vi "DIO Block Write.vi"(7 "Divisor":u16, 8 "DIR":bool, 9 "OUT":bool, 10 "DMA FIFO In":refnum<k21>="A.DO1 DMA", 11 "DIO Refnum":refnum<k21>="ConnectorA/DIO0") -> (1 "Timed Out?":bool, 3 "IN":bool)   [LabVIEW 2014]
uses:
  <vilib>/rvi/eio/common/nirviEmuReportErrorAndStop.vi
  <vilib>/rvi/interface/RandomDataEmulation/niFpgaRandomDataHandleErrors.vi
  <vilib>/rvi/Emulation/niFpgaProcessEmulError.vi
  <vilib>/rvi/FIFO/Fifo_Resource/nirvififoEmulationSetSize.vi
  <vilib>/rvi/DataTransferAndStorage/Container/Common/niFpgaContainerGetUniqueNameForEmu.vi
  <vilib>/rvi/FIFO/Fifo_Resource/nirviFifoEmulationQueueMgr.vi
  <instcachedir>/0/nirviFifoEmulationQueueMgr_E5CAEC123FF24DC58D834DCA3CDAA9B5.lvgen/nirviFifoEmulationQueueMgr_E5CAEC123FF24DC58D834DCA3CDAA9B5_001.vi
  <vilib>/rvi/Emulation/niFpgaEmulationIsFPGAContextNoSignature.vi
  <vilib>/rvi/errors/nirviReportUnexpectedCaseInternalError.vi
  <vilib>/rvi/errors/nirviReportUnexpectedCaseInternalError (U32).vi
  <vilib>/rvi/occurrence/nirviWaitOnOccurrenceBase.vi
  <vilib>/rvi/FIFO/Fifo_Resource/nirvififoEmulationReleaseLock.vi
  <vilib>/rvi/FIFO/Fifo_Resource/nirvififoEmulationObtainLock.vi
  <vilib>/rvi/FIFO/Fifo_Resource/nirvififoEmulationCreateLock.vi
  <vilib>/rvi/errors/niFpgaSetErrorForExecOnDevCompSimple.vi
  <vilib>/rvi/Emulation/niFpgaSctlEmulationGetInTimedLoop.vi
  <vilib>/rvi/FIFO/Fifo_Resource/nirvififoEmulationDetermineInputValidOut.vi
  <vilib>/rvi/DataTransferAndStorage/Container/Common/niFpgaContainerExecOnDevCompGetState.vi
  <vilib>/rvi/DataTransferAndStorage/Container/XNode/niFpgaContainer.xnode
  <vilib>/rvi/FIFO/Fifo_Resource/niFpgaFifoEmulationRefIn.vi
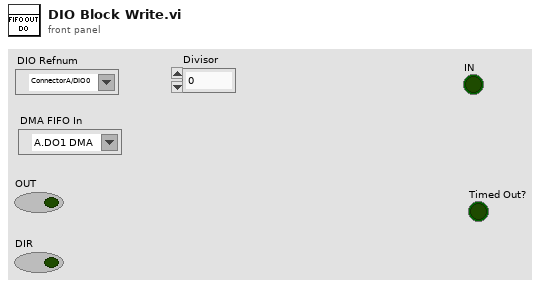
[diagram p1: front panel]
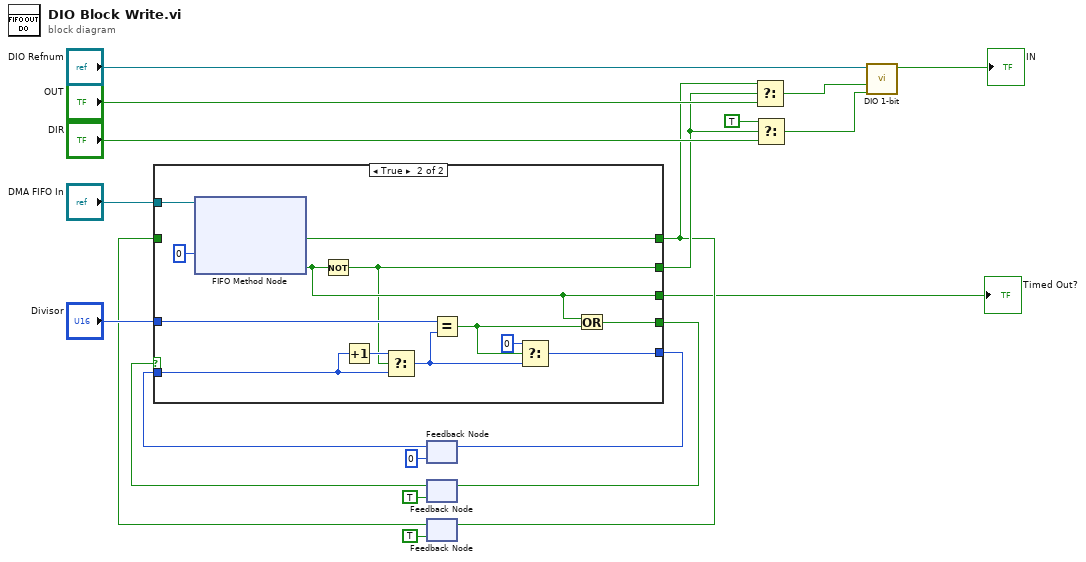
[diagram p0: block diagram]
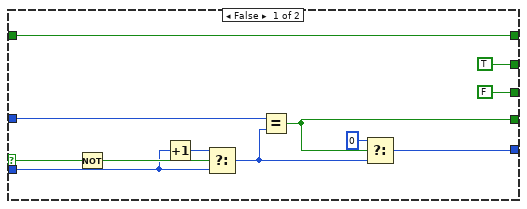
[diagram p2: hidden frame]
diagram:
  n1 = feedback #1(u16 0 ("t")) -> (w1:u16)
  n2 = feedback #2(TRUE ("Timed Out?")) -> (w11:bool)
  n3 = feedback #3(TRUE ("Timed Out?")) -> (w6:bool)
  n4 = case shown="True" w11 {
    selector: w11 -> [w32 _]
    tunnel: [w29 w44] -> w7
    tunnel: [TRUE w35] -> w9
    tunnel: "Divisor" -> [w24 w36]
    tunnel: [w21 w43] -> w12
    tunnel: [FALSE ("Timed Out?") w42] -> w5
    tunnel: w6 -> [w29 _]
    tunnel: "DMA FIFO In" -> [_ w41]
    tunnel: [w22 w34] -> w2
    tunnel: w1 -> [w23 w33]
    frame False {
      n5 = Not(x=w32) -> (.not. x?=w25:bool)
      n6 = Increment(x=w23) -> (x+1=w28:u16)
      n7 = Select(t=w28, s=w25, f=w23) -> (s? t:f=w26:u16)
      n8 = Equal?(x=w24, y=w26) -> (x = y?=w21:bool)
      n9 = Select(t=u16 0, s=w21, f=w26) -> (s? t:f=w22:u16)
    }
    frame True {
      n10 = xnode ("FIFO Method Node")("Timeout"=0, "FIFO In"=w41) -> ("Element"=w44:bool, "Timed Out?"=w42:bool)  [unwired: 1 out]
      n11 = Not(x=w42) -> (.not. x?=w35:bool)
      n12 = Increment(x=w33) -> (x+1=w40:u16)
      n13 = Select(t=w40, s=w35, f=w33) -> (s? t:f=w38:u16)
      n14 = Equal?(x=w36, y=w38) -> (x = y?=w37:bool)
      n15 = Select(t=u16 0, s=w37, f=w38) -> (s? t:f=w34:u16)
      n16 = Or(x=w42, y=w37) -> (x .or. y?=w43:bool)
    }
  }
  "Timed Out?" <- w5
  n17 = feedback-in #1(w2) -> ()
  n18 = feedback-in #2(w12) -> ()
  n19 = feedback-in #3(w7) -> ()
  n20 = Select(t=w7, s=w9, f="OUT") -> (s? t:f=w17:bool)
  n21 = Select(t=TRUE ("Flag"), s=w9, f="DIR") -> (s? t:f=w14:bool)
  n22 = call "DIO 1-bit.vi"("DIR"=w14, "OUT"=w17, "DIO Refnum"="DIO Refnum") -> ("IN"=→"IN":bool)  [unwired: 8 in]
